vi "modbus通讯.vi"(9 "工步号":refnum<queue>, 10 "变更完成反馈":refnum<queue>, 11 "变更允许":refnum<queue>) -> ()   [LabVIEW 2013]
uses:
  <vilib>/Platform/TimedLoop/XDataNode/timing_clust.ctl
  <vilib>/Platform/TimedLoop/XDataNode/nitl_modes.ctl
  <vilib>/Platform/TimedLoop/XDataNode/wakeup.ctl
  <vilib>/NI Modbus.llb/MB Ethernet Master Query Write Single Register (poly).vi
  <vilib>/Platform/TimedLoop/XDataNode/XDataNode.xnode
  <vilib>/Platform/TimedLoop/XDataNode/XDNodeRunTimeDep.lvlib
panel:
  out "status":bool
  out "TCP报警":errorcluster caption="错误输出"
  in  "工步号2":u16
  out "工步变更允许":bool
  out "错误输出":errorcluster
  out "TCPIP":refnum<k5>
  out "错误输出 2":errorcluster caption="错误输出"
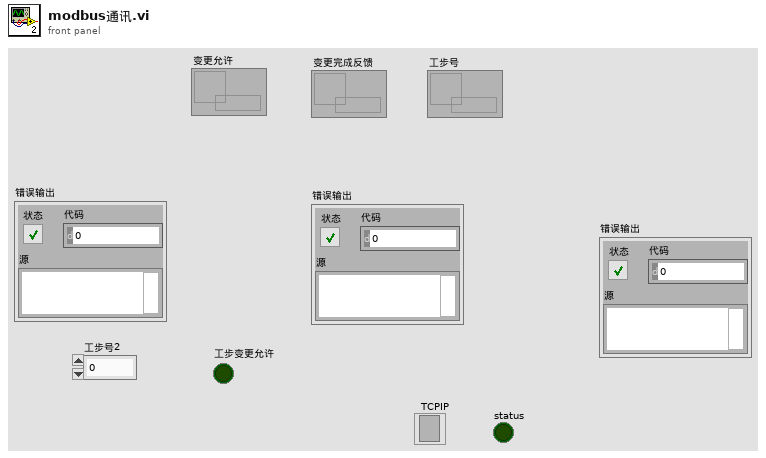
[diagram p1: front panel]
types:
  T1 = typedef "XDNodeRunTimeDep.lvlib/timing_clust.ctl" = cluster{"Expected End [f-1]":u64, "Actual End [f-1]":u64, "Finished Late? [f-1]":bool, "Expected End [i-1]":u64, "Actual End [i-1]":u64, "Finished Late? [i-1]":bool, "Expected Start [i]":u64, "Actual Start [i]":u64, "Expected Start [f]":u64, "Actual Start [f]":u64, "Source Name":string, "Structure Name":string, "Period":i64, "Deadline":i64, "Offset":i64, "Start":i64, "Priority":i32, "Timeout":i32, "Mode":T2, "Wakeup Reason":T3, "Error":errorcluster, "Source Type":string, "Secondary Source Type":string, "Global End Time":u64, "Global Start Time":u64, "Frame Duration":u64, "Iteration Duration":u64, "Assigned CPU":i32, "I/O Scan Engine Mode":u32}
  T2 = typedef "XDNodeRunTimeDep.lvlib/nitl_modes.ctl" = enum32{"No Change", "Process missed periods, maintain original phase", "Discard missed periods, maintain original phase", "Process missed periods, ignore original phase", "Discard missed periods, ignore original phase"}
  T3 = typedef "XDNodeRunTimeDep.lvlib/wakeup.ctl" = enum32{"Normal", "Aborted", "Asynchronous wakeup", "Timing source error", "Timed loop error", "Timeout"}
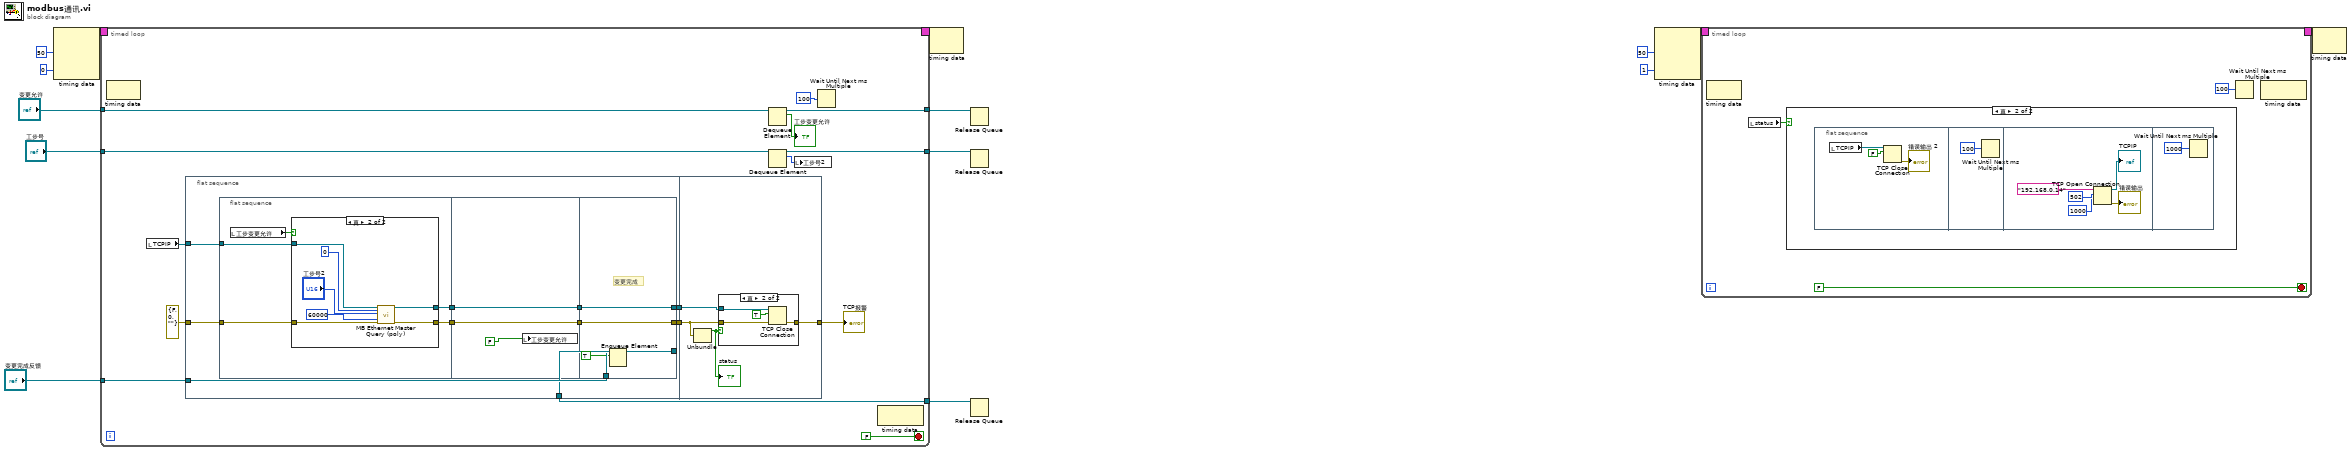
[diagram p0: block diagram]
diagram:
  n1 = node-c288(i64 50 ("周期"), 0 ("处理器")) -> (w10:T1)  [unwired: 2 in]
  n2 = timed-loop {
    timing: w10 -> [_]
    timing-out: [_] -> w9
    tunnel: "变更允许" -> [w22]
    tunnel: "工步号" -> [w20]
    tunnel: "变更完成反馈" -> [w18]
    tunnel: [w17] -> w3
    tunnel: [w16] -> w2
    tunnel: [w15] -> w1
    stop <- FALSE stop-if-true
    n3 = node-c288() -> ()  [unwired: 1 in, 1 out]
    n4 = local read "TCPIP"() -> (w24:refnum<k5>)
    n5 = flat-sequence {
      tunnel: [w40] -> w27
      tunnel: [w41] -> w26
      tunnel: errorcluster {"status"=FALSE, "code"=0, "source"=""} ("error out") -> [w39]
      tunnel: w24 -> [w38]
      tunnel: w18 -> [w37]
      tunnel: [w36] -> w16
      tunnel: w27 -> [w66]
      tunnel: [w65] -> w28
      tunnel: w26 -> [w64]
      frame #0 {
        n6 = flat-sequence {
          tunnel: w38 -> [w45]
          tunnel: w39 -> [w44]
          tunnel: [w43] -> w35
          tunnel: [w42] -> w33
          tunnel: w35 -> [w58]
          tunnel: [w58] -> w34
          tunnel: w33 -> [w57]
          tunnel: [w57] -> w32
          tunnel: w34 -> [w63]
          tunnel: w32 -> [w62]
          tunnel: [w63] -> w41
          tunnel: [w62] -> w40
          tunnel: w37 -> [w61]
          tunnel: [w59] -> w36
          frame #0 {
            n7 = local read "工步变更允许"() -> (w46:bool)
            n8 = case shown="真" w46 {
              tunnel: w45 -> [w48 w53]
              tunnel: [w48 w52] -> w43
              tunnel: w44 -> [w47 w51]
              tunnel: [w47 w50] -> w42
              frame False {
              }
              frame True {
                n9 = call-poly <vilib>:"MB Ethernet Master Query (poly).vi"("TCP Connection Refnum in"=w53, "Address"=u16 0, "Register"="工步号2", "Timeout"=u32 60000, "error in"=w51) -> ("TCP Connection Refnum (dup)"=w52:refnum<k5>, "error out"=w50:errorcluster)  [unwired: 12 in, 1 out]
              }
            }
          }
          frame #1 {
            n10 = local write "工步变更允许"(FALSE ("工步变更允许")) -> ()
          }
          frame #2 {
            # "变更完成"
            n11 = Enqueue Element(queue=w61, element=TRUE ("工步变更允许")) -> (queue out=w59:refnum<queue>)  [unwired: 2 in, 2 out]
          }
        }
      }
      frame #1 {
        n12 = Unbundle(w66) -> ("status"=w67:bool)  [unwired: 2 out]
        "status" <- w67
        n13 = case shown="真" w67 {
          tunnel: w64 -> [_ w72]
          tunnel: w66 -> [w68 w70]
          tunnel: [w68 w69] -> w65
          frame False {
          }
          frame True {
            n14 = TCP Close Connection(connection ID=w72, abort (F)=TRUE ("中止(F)"), error in (no error)=w70) -> (error out=w69:errorcluster)  [unwired: 1 out]
          }
        }
      }
    }
    n15 = Dequeue Element(queue=w22) -> (queue out=w17:refnum<queue>, element=→"工步变更允许":bool)  [unwired: 2 in, 2 out]
    n16 = Dequeue Element(queue=w20) -> (queue out=w15:refnum<queue>, element=w19:i32)  [unwired: 2 in, 2 out]
    n17 = local write "工步号2"(w19) -> ()
    n18 = Wait Until Next ms Multiple(millisecond multiple=u32 100 ("毫秒倍数")) -> ()  [unwired: 1 out]
    n19 = node-c288() -> ()  [unwired: 1 in, 1 out]
    "TCP报警" <- w28
  }
  n20 = node-c288(w9) -> ()  [unwired: 1 out]
  n21 = Release Queue(queue=w3) -> ()  [unwired: 2 in, 3 out]
  n22 = Release Queue(queue=w1) -> ()  [unwired: 2 in, 3 out]
  n23 = Release Queue(queue=w2) -> ()  [unwired: 2 in, 3 out]
  n24 = node-c288(i64 50 ("周期"), 1 ("处理器")) -> (w14:T1)  [unwired: 2 in]
  n25 = timed-loop {
    timing: w14 -> [_]
    timing-out: [_] -> w13
    stop <- FALSE stop-if-true
    n26 = node-c288() -> ()  [unwired: 1 in, 1 out]
    n27 = local read "status"() -> (w75:bool)
    n28 = case shown="真" w75 {
      frame False {
      }
      frame True {
        n29 = flat-sequence {
          frame #0 {
            n30 = local read "TCPIP"() -> (w79:refnum<k5>)
            n31 = TCP Close Connection(connection ID=w79, abort (F)=FALSE ("中止(F)")) -> (error out=→"错误输出 2":errorcluster)  [unwired: 1 in, 1 out]
          }
          frame #1 {
            n32 = Wait Until Next ms Multiple(millisecond multiple=u32 100 ("毫秒倍数")) -> ()  [unwired: 1 out]
          }
          frame #2 {
            n33 = TCP Open Connection(address="192.168.0.14" ("地址"), remote port or service name=u16 502 ("远程端口或服务名称"), timeout ms (60000)=1000 ("超时毫秒(60000)")) -> (connection ID=→"TCPIP":refnum<k5>, error out=→"错误输出":errorcluster)  [unwired: 2 in]
          }
          frame #3 {
            n34 = Wait Until Next ms Multiple(millisecond multiple=u32 1000 ("毫秒倍数")) -> ()  [unwired: 1 out]
          }
        }
      }
    }
    n35 = Wait Until Next ms Multiple(millisecond multiple=u32 100 ("毫秒倍数")) -> ()  [unwired: 1 out]
    n36 = node-c288() -> ()  [unwired: 1 in, 1 out]
  }
  n37 = node-c288(w13) -> ()  [unwired: 1 out]
